vi "CLSUIP_IsOldVIOwnedByInterface.vi"(11 "VIRetooler in":refnum<class "VIRetooler.lvclass">) -> (3 "is interface":bool)   [LabVIEW 2021, in "MemberVICreation.lvlib" / "VIRetooler.lvclass"]
uses:
  <resource>/Framework/Providers/LVClassLibrary/NewAccessors/VIRetooler/VIRetooler.lvclass
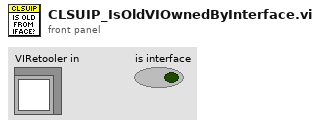
[diagram p1: front panel]
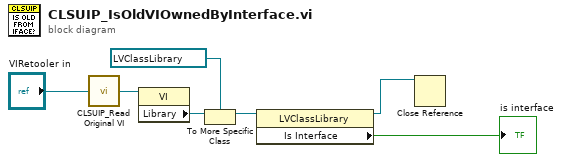
[diagram p0: block diagram]
diagram:
  n1 = call <resource>:"CLSUIP_Read Original VI.vi"("VIRetooler.lvclass in"="VIRetooler in") -> ("Original VI"=w6:refnum<vi>)
  n2 = property class="VI"(reference=w6) -> ("Library"=w5:refnum<vi>)  [unwired: 1 in, 2 out]
  n3 = To More Specific Class(target class=refnum<vi> refnum ("Library"), reference=w5) -> (specific class reference=w3:refnum<vi>)  [unwired: 1 in, 1 out]
  n4 = property class="LVClassLibrary"(reference=w3) -> (reference out=w1:refnum<vi>, "Is Interface"=→"is interface":bool)  [unwired: 1 in, 1 out]
  n5 = Close Reference(reference=w1) -> ()  [unwired: 1 in, 1 out]
